vi "BASE_Login Screen.vi"(8 "Error In":errorcluster, 10 "Password":string, 11 "User Name":string(combo)) -> (0 "error out":errorcluster, 1 "Level":i32, 2 "Login Done":bool, 3 "User Name Out":string(combo))   [LabVIEW 2017]
uses:
  <vilib>/Utility/config.llb/Read Key (String).vi
  <vilib>/Utility/config.llb/Read Key (I32).vi
  <vilib>/Utility/config.llb/NI_LVConfig.lvlib
panel:
  in  "Cancel":bool
  in  "OK Button":bool
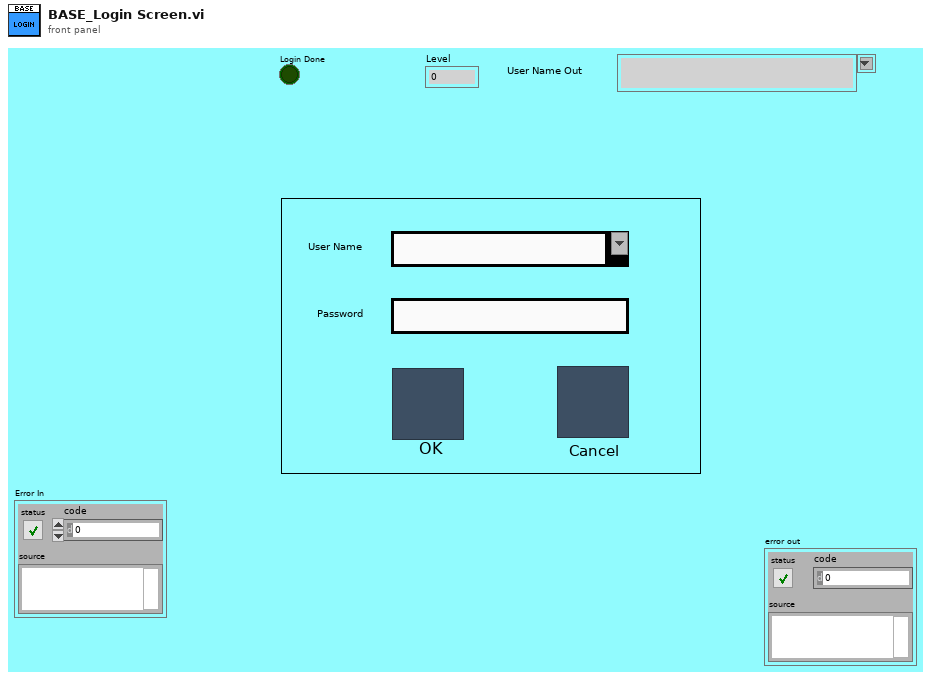
[diagram p1: front panel]
types:
  T1 = enum32{"invalid app kind", "Development System", "Run Time System", "Student Edition", "Embedded LabVIEW", "Evaluation", "Custom"}
  T2 = typedef "NI_LVConfig.lvlib/Config Data RefNum.ctl" = refnum<k1>
  T3 = enum32{"Invalid", "Standard", "Closed", "Hidden", "Minimized", "Maximized"}
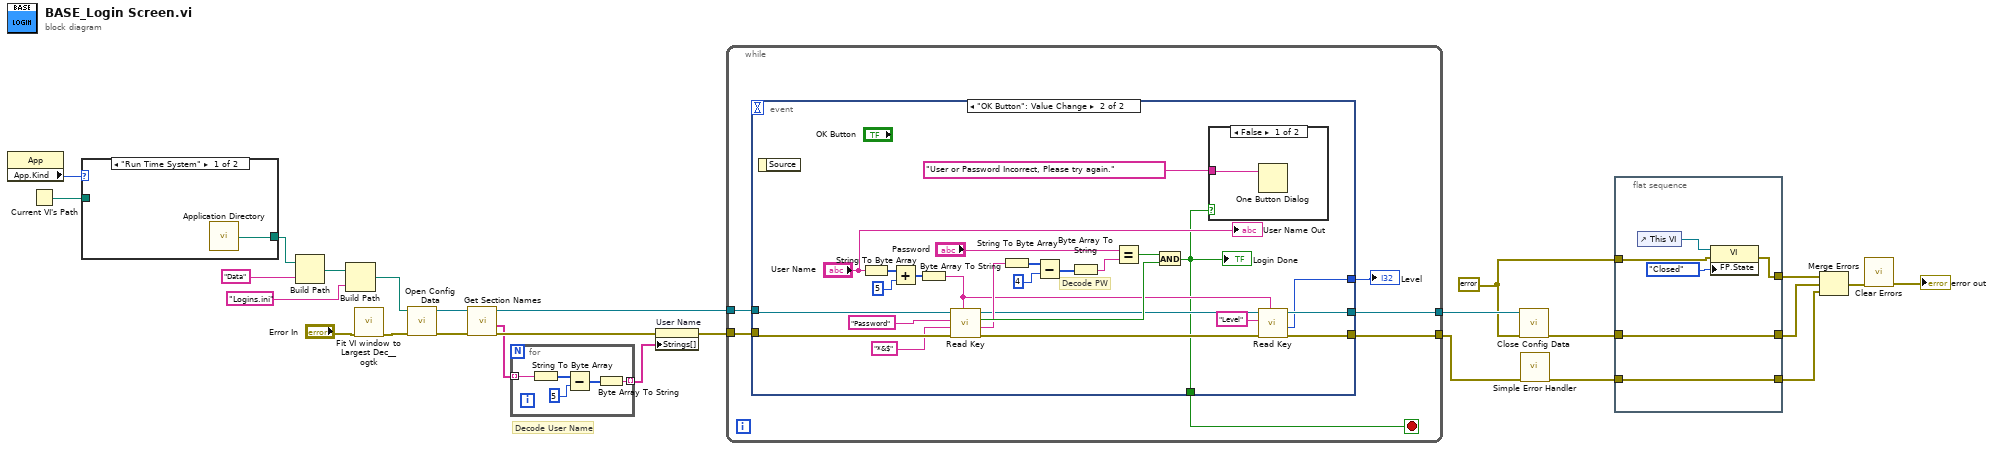
[diagram p0: block diagram]
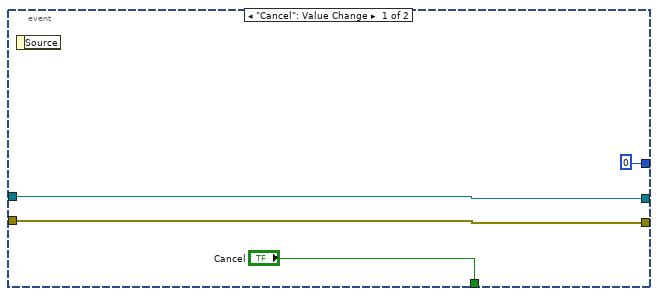
[diagram p2: hidden frame]
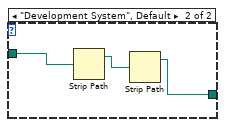
[diagram p4: hidden frame]
diagram:
  w17 = errorcluster {"status"=FALSE, "code"=0, "source"=""} ("error in (no error)")
  # "Decode User Name"
  n1 = property class="App"() -> ("App.Kind"=w25:T1)  [unwired: 2 in, 2 out]
  n2 = Current VI's Path() -> (path=w26:path)
  n3 = case shown="\"Run Time System\"" w25 {
    tunnel: w26 -> [_ w29]
    tunnel: [w27 w28] -> w23
    frame "Run Time System" {
      n4 = call <vilib>:"Application Directory.vi"() -> ("Application Directory"=w27:path)
    }
    frame "Development System", Default {
      n5 = Strip Path(path=w29) -> (stripped path=w30:path)  [unwired: 1 out]
      n6 = Strip Path(path=w30) -> (stripped path=w28:path)  [unwired: 1 out]
    }
  }
  n7 = Build Path(base path=w23, name or relative path="Data") -> (appended path=w24:path)
  n8 = Build Path(base path=w24, name or relative path="Logins.ini") -> (appended path=w22:path)
  n9 = call <userlib>:"Fit VI window to Largest Dec__ogtk.vi"("error in (no error)"="Error In") -> ("error out"=w1:errorcluster)  [unwired: 5 in, 1 out]
  n10 = call <vilib>:"Open Config Data.vi"("error in (no error)"=w1, "configuration file path"=w22) -> ("error out"=w8:errorcluster, "refnum"=w9:T2)  [unwired: 7 in, 1 out]
  n11 = call <vilib>:"Get Section Names.vi"("error in (no error)"=w8, "refnum"=w9) -> ("error out"=w6:errorcluster, "section names"=w4:string[], "refnum out"=w7:T2)  [unwired: 7 in]
  n12 = for {
    tunnel: w4 -> [w35] mode=indexing
    tunnel: [w31] -> w3 mode=indexing
    n13 = String To Byte Array(string=w35) -> (unsigned byte array=w34:u8[])
    n14 = Subtract(x=w34, y=u8 5) -> (x-y=w32:u8[])
    n15 = Byte Array To String(unsigned byte array=w32) -> (string=w31:string)
  }
  n16 = property on="User Name" class="CmbBox"(error in=w6, "Strings[]"=w3) -> (error out=w5:errorcluster)  [unwired: 1 in, 1 out]
  n17 = while {
    tunnel: [w40] -> w19
    tunnel: w7 -> [w39]
    tunnel: [w38] -> w18
    tunnel: w5 -> [w37]
    stop <- w41 stop-if-true
    n18 = event shown="[1] \"OK Button\": Value Change" {
      selector: _ -> [_ _]
      dyn-events: _ -> [_ _]
      timeout: _ -> [_ _]
      tunnel: ["Cancel" w47] -> w41
      tunnel: [w44 w51] -> w40
      tunnel: w39 -> [w44 w70]
      tunnel: [w43 w50] -> w38
      tunnel: w37 -> [w43 w69]
      tunnel: [0 ("value") w48] -> w36
      event "Cancel": Value Change {
        n19 = event-data() -> ()  [unwired: 1 in, 1 out]
      }
      event "OK Button": Value Change {
        # "Decode PW"
        n20 = event-data() -> ()  [unwired: 1 in, 1 out]
        n21 = String To Byte Array(string="User Name") -> (unsigned byte array=w58:u8[])
        n22 = Add(x=w58, y=u8 5) -> (x+y=w56:u8[])
        n23 = Byte Array To String(unsigned byte array=w56) -> (string=w54:string)
        n24 = call-poly <vilib>:"Read Key.vi"("section"=w54, "error in (no error)"=w69, "default value"="*&$", "key"="Password", "refnum"=w70) -> ("error out"=w53:errorcluster, "value"=w63:string, "found?"=w65:bool, "refnum out"=w52:T2)  [unwired: 3 in]
        n25 = String To Byte Array(string=w63) -> (unsigned byte array=w62:u8[])
        n26 = Subtract(x=w62, y=u8 4) -> (x-y=w60:u8[])
        n27 = Byte Array To String(unsigned byte array=w60) -> (string=w59:string)
        n28 = Equal?(x="Password", y=w59) -> (x = y?=w66:bool)
        n29 = And(x=w66, y=w65) -> (x .and. y?=w47:bool)
        "Login Done" <- w47
        n30 = case shown="False" w47 {
          tunnel: "User or Password Incorrect, Please try again." -> [w71 _]
          frame False {
            n31 = One Button Dialog(message=w71) -> ()  [unwired: 1 in, 1 out]
          }
          frame True {
          }
        }
        n32 = call-poly <vilib>:"Read Key.vi"("section"=w54, "error in (no error)"=w53, "key"="Level", "refnum"=w52) -> ("error out"=w50:errorcluster, "value"=w48:i32, "refnum out"=w51:T2)  [unwired: 4 in, 1 out]
        "User Name Out" <- "User Name"
      }
    }
    "Level" <- w36
  }
  n33 = call <vilib>:"Close Config Data.vi"("error in (no error)"=w17, "refnum"=w19) -> ("error out"=w12:errorcluster)  [unwired: 8 in, 1 out]
  n34 = call <vilib>:"Simple Error Handler.vi"("error in (no error)"=w18) -> ("error out"=w10:errorcluster)  [unwired: 4 in, 4 out]
  n35 = flat-sequence {
    tunnel: w17 -> [w75]
    tunnel: [w74] -> w16
    tunnel: [w73] -> w13
    tunnel: w12 -> [w73]
    tunnel: [w72] -> w11
    tunnel: w10 -> [w72]
    frame #0 {
      n36 = control-ref of="This VI"() -> (w77:refnum<vi>)
      n37 = property class="VI"(reference=w77, error in=w75, "FP.State"=T3."Closed" ("Front Panel Window:State")) -> (error out=w74:errorcluster)  [unwired: 1 out]
    }
  }
  n38 = Merge Errors(w16, w13, w11) -> (w15:errorcluster)
  n39 = call <vilib>:"Clear Errors.vi"("error in (no error)"=w15) -> ("error out"=→"error out":errorcluster)  [unwired: 5 in, 1 out]
